vi "TreeNode Make Segment.vi"(0 "TreeNode DVR in":refnum<data-value>, 1 "Start":refnum<data-value>, 2 "End":refnum<data-value>, 3 "Dimension":refnum<data-value>, 4 "Data":refnum<data-value>, 5 "error in (no error)":errorcluster) -> (14 "TreeNode DVR out":refnum<data-value>, 19 "error out":errorcluster)   [LabVIEW 2012, in "MDSplus.lvlib"]
doc: "Initializes and fills a new segment."
uses:
  <vilib>/MDSplus/Library/MDSplus.lvlib
  <vilib>/MDSplus/Classes/Data_Class/TreeNode_Class/TreeNode.lvclass
  <vilib>/MDSplus/Classes/Data_Class/Data.lvclass
  <vilib>/MDSplus/Classes/Data_Class/Array_Class/Array.lvclass
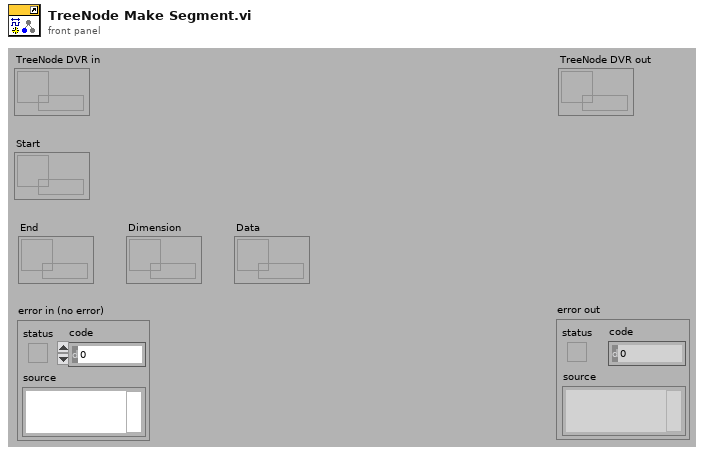
[diagram p1: front panel]
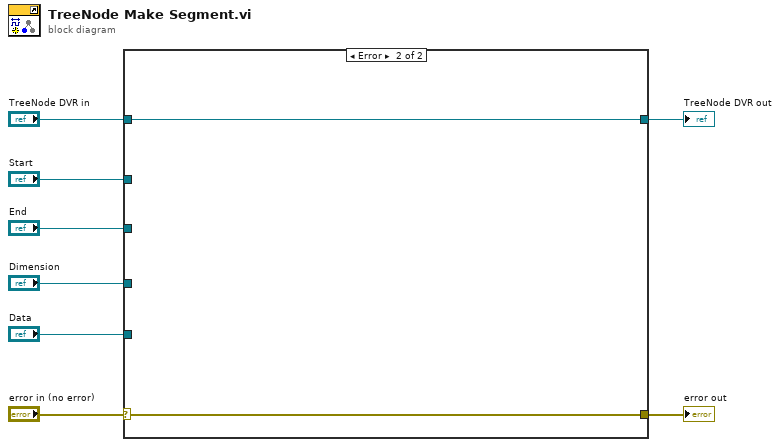
[diagram p0: block diagram]
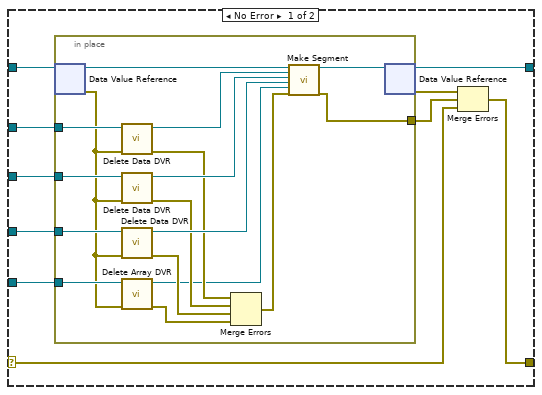
[diagram p2: hidden frame]
diagram:
  n1 = case shown="Error" "error in (no error)" {
    selector: "error in (no error)" -> [w11 w36]
    tunnel: [w10 w36] -> w8
    tunnel: [w9 w37] -> w6
    tunnel: "Start" -> [w18 _]
    tunnel: "End" -> [w17 _]
    tunnel: "Dimension" -> [w16 _]
    tunnel: "Data" -> [w15 _]
    tunnel: "TreeNode DVR in" -> [w14 w37]
    frame No Error {
      n2 = in-place {
        in-place-border: w18 -> [w35]
        in-place-border: w17 -> [w34]
        in-place-border: w16 -> [w33]
        in-place-border: w15 -> [w25]
        in-place-border: [w19] -> w12
        n3 = in-place-dvr #1(w14) -> (w23:refnum<class "TreeNode.lvclass">, w22:errorcluster)
        n4 = call <vilib>:"Delete Data DVR.vi"("error in (no error)"=w22, "Data DVR in"=w35) -> ("error out"=w27:errorcluster, "Data out"=w32:refnum<class "Data.lvclass">)  [unwired: 8 in]
        n5 = call <vilib>:"Delete Data DVR.vi"("error in (no error)"=w22, "Data DVR in"=w34) -> ("error out"=w28:errorcluster, "Data out"=w31:refnum<class "Data.lvclass">)  [unwired: 8 in]
        n6 = call <vilib>:"Delete Data DVR.vi"("error in (no error)"=w22, "Data DVR in"=w33) -> ("error out"=w29:errorcluster, "Data out"=w30:refnum<class "Data.lvclass">)  [unwired: 8 in]
        n7 = call <vilib>:"Delete Array DVR.vi"("error in (no error)"=w22, "Array DVR in"=w25) -> ("error out"=w24:errorcluster, "Array out"=w21:refnum<class "Array.lvclass">)  [unwired: 8 in]
        n8 = Merge Errors(w27, w28, w29, w24) -> (w26:errorcluster)
        n9 = call-dynamic "Make Segment.vi"("TreeNode in"=w23, "Start"=w32, "End"=w31, "Dimension"=w30, "Data"=w21, "error in (no error)"=w26) -> ("TreeNode out"=w20:refnum<class "TreeNode.lvclass">, "error out"=w19:errorcluster)  [unwired: 12 in]
        n10 = in-place-dvr #1(w20) -> (w9:refnum<data-value>, w13:errorcluster)
      }
      n11 = Merge Errors(w13, w12, w11) -> (w10:errorcluster)
    }
    frame Error {
    }
  }
  "error out" <- w8
  "TreeNode DVR out" <- w6
